vi "configure.vi"(8 "error in (no error)":errorcluster, 9 "Value":i32, 10 "ILC":refnum<class "ILC.lvclass">, 11 "IConfigureILCStrategy in":refnum<class "ConfigureILCROTStrategy.lvclass">) -> (0 "error out":errorcluster, 3 "IConfigureILCStrategy out":refnum<class "ConfigureILCROTStrategy.lvclass">)   [LabVIEW 2015, in "ConfigureILCROTStrategy.lvclass"]
uses:
  ConfigureILCROTStrategy.lvclass
  <userlib>/Common/ILC/ILC/ILC.lvclass
  <userlib>/Common/ILC/ILC/ILC.lvclass/ILC.ctl
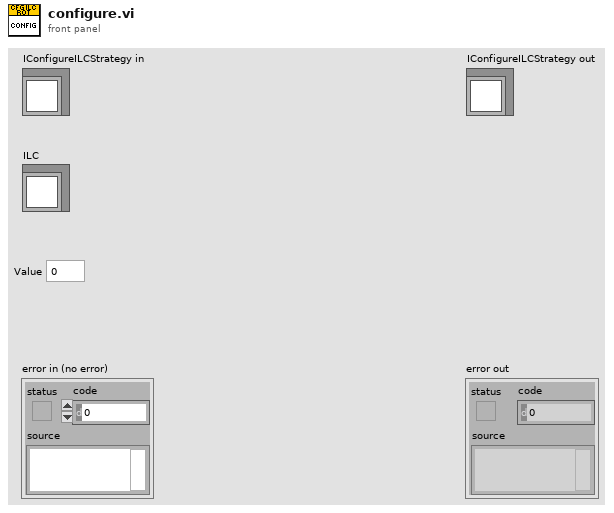
[diagram p1: front panel]
types:
  T1 = typedef "ILCCommon.lvlib/ILCTypedefs.lvlib/OutputData.ctl" = cluster{"Step & Direction":i16, "Blower RPM":u8, "PWM (SSR)":u8, "Ch1":u16, "Ch2":u16, "Ch3":u16, "Ch4":u16}
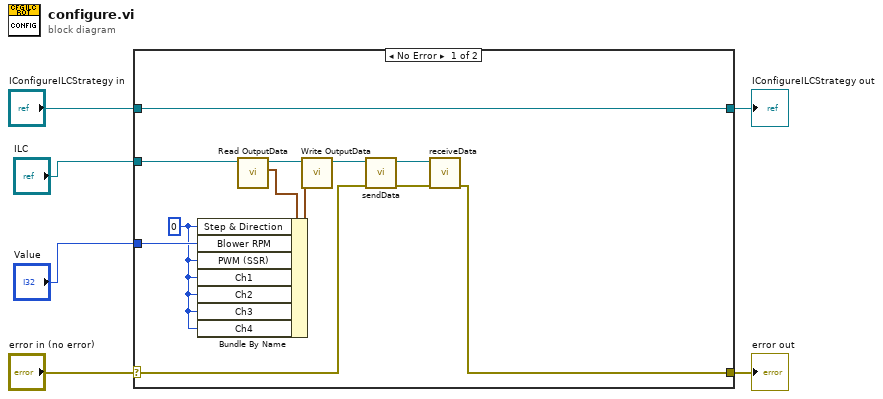
[diagram p0: block diagram]
diagram:
  n1 = case shown="No Error" "error in (no error)" {
    selector: "error in (no error)" -> [w10 w20]
    tunnel: [w8 w20] -> w5
    tunnel: [w18 w19] -> w3
    tunnel: "IConfigureILCStrategy in" -> [w18 w19]
    tunnel: "ILC" -> [w17 _]
    tunnel: "Value" -> [w15 _]
    frame No Error {
      w7 = i16 0 ("Step & Direction")
      n2 = call <userlib>:"Read OutputData.vi"("ILC in"=w17) -> ("OutputData"=w16:T1, "ILC out"=w13:refnum<class "ILC.lvclass">)  [unwired: 9 in]
      n3 = Bundle By Name(cluster=w16, "Step & Direction"=w7, "Blower RPM"=w15, "PWM (SSR)"=w7, "Ch1"=w7, "Ch2"=w7, "Ch3"=w7, "Ch4"=w7) -> (w14:T1)
      n4 = call <userlib>:"Write OutputData.vi"("OutputData"=w14, "ILC in"=w13) -> ("ILC out"=w12:refnum<class "ILC.lvclass">)  [unwired: 9 in]
      n5 = call <userlib>:"sendData.vi"("error in (no error)"=w10, "ILC in"=w12) -> ("error out"=w9:errorcluster, "ILC out"=w11:refnum<class "ILC.lvclass">)  [unwired: 8 in]
      n6 = call <userlib>:"receiveData.vi"("error in (no error)"=w9, "ILC in"=w11) -> ("error out"=w8:errorcluster)  [unwired: 8 in, 1 out]
    }
    frame Error {
    }
  }
  "error out" <- w5
  "IConfigureILCStrategy out" <- w3
